vi "Read clientID.vi"(8 "error in (no error)":errorcluster, 11 "mqtt in":refnum<class "MQTT Client.lvclass">) -> (0 "error out":errorcluster, 2 "clientID":string, 3 "mqtt out":refnum<class "MQTT Client.lvclass">)   [LabVIEW 2020, in "MQTT Client.lvclass"]
uses:
  MQTT Client.lvclass
  MQTT Client.lvclass/MQTT Client.ctl
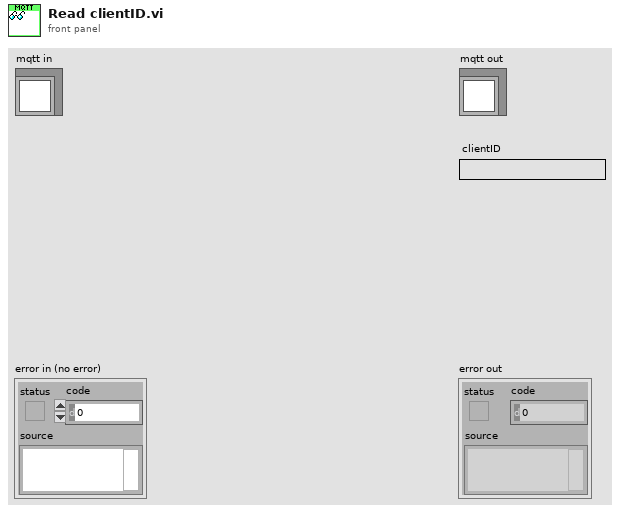
[diagram p1: front panel]
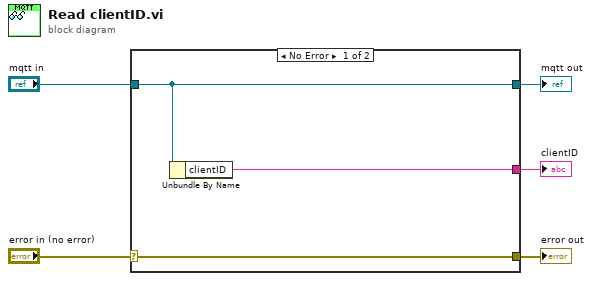
[diagram p0: block diagram]
diagram:
  n1 = case shown="No Error" "error in (no error)" {
    selector: "error in (no error)" -> [w8 w9]
    tunnel: [w8 w9] -> w4
    tunnel: [w7 w10] -> w2
    tunnel: "mqtt in" -> [w7 w10]
    tunnel: [w6 _] -> w1
    frame No Error {
      n2 = Unbundle By Name(w7) -> ("clientID"=w6:string)
    }
    frame Error {
    }
  }
  "error out" <- w4
  "mqtt out" <- w2
  "clientID" <- w1
